vi "Arduino_DHT22_sensor.vi"() -> ()   [LabVIEW 2013]
uses:
  <vilib>/Instr/_visa.llb/VISA Configure Serial Port (Instr).vi
panel:
  out "Waveform Chart 2":dbl[](graph)
  out "Dew Point Temp (C)":dbl
  out "Temp (C)":dbl
  out "Waveform Chart":dbl[](graph)
  out "Humidity (%)":dbl
  in  "stop":bool
  # "Arduino Temperature and Humidity Sensing"
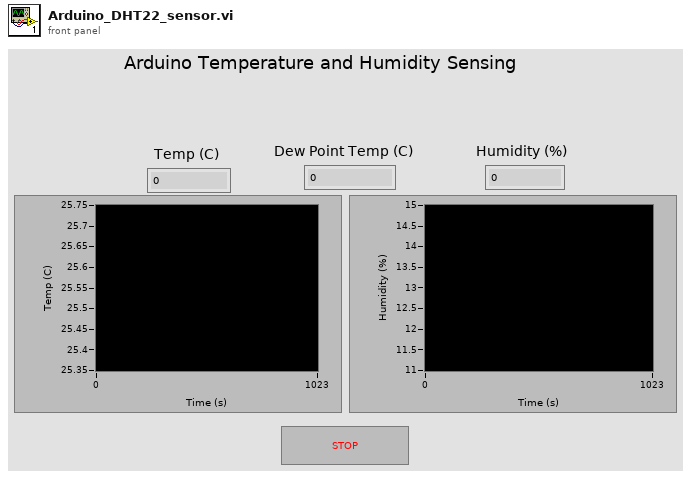
[diagram p1: front panel]
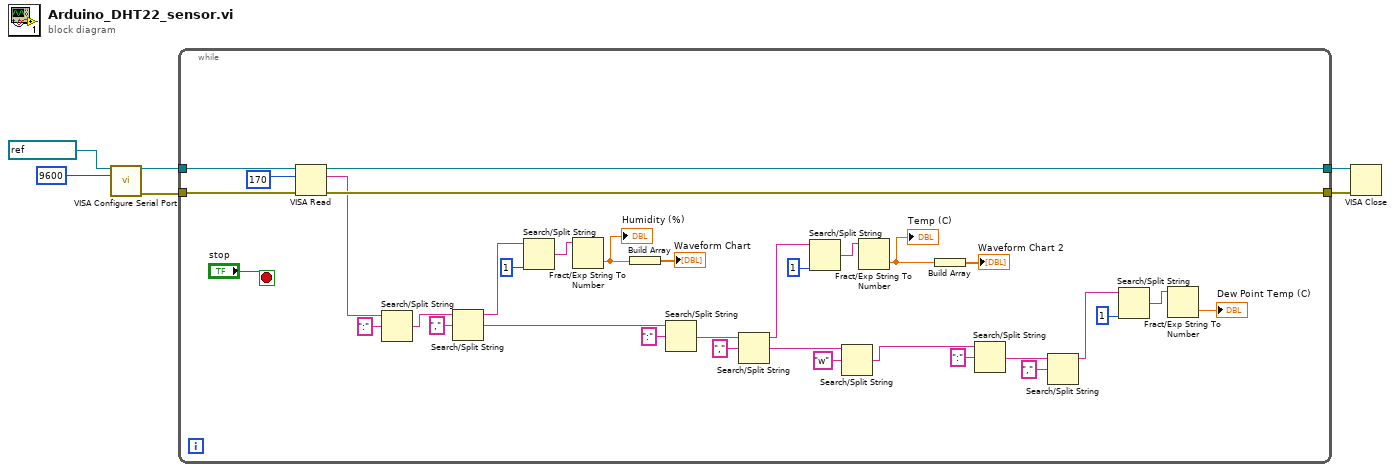
[diagram p0: block diagram]
diagram:
  n1 = call-poly "VISA Configure Serial Port"("VISA resource name"=refnum<visa-resource-name> "COM12", "baud rate (9600)"=u32 9600) -> ("VISA resource name out"=w3:refnum<visa-resource-name>, "error out"=w4:errorcluster)  [unwired: 12 in]
  n2 = while {
    tunnel: w3 -> [w36]
    tunnel: w4 -> [w35]
    tunnel: [w39] -> w6
    tunnel: [w38] -> w5
    stop <- "stop" stop-if-true
    n3 = VISA Read(VISA resource name=w36, byte count=u32 170, error in (no error)=w35) -> (VISA resource name out=w39:refnum<visa-resource-name>, read buffer=w34:string, error out=w38:errorcluster)  [unwired: 1 out]
    n4 = Search/Split String(string=w34, search string/char (-)=":") -> (match + rest of string=w31:string)  [unwired: 1 in, 2 out]
    n5 = Search/Split String(string=w31, search string/char (-)=",") -> (substring before match=w26:string, match + rest of string=w30:string)  [unwired: 1 in, 1 out]
    n6 = Search/Split String(string=w26, offset (0)=1) -> (match + rest of string=w24:string)  [unwired: 1 in, 2 out]
    n7 = Fract/Exp String To Number(string=w24) -> (number=w23:dbl)  [unwired: 3 in, 1 out]
    "Humidity (%)" <- w23
    n8 = Build Array(w23) -> (→"Waveform Chart":dbl[])
    n9 = Search/Split String(string=w30, search string/char (-)=":") -> (match + rest of string=w27:string)  [unwired: 1 in, 2 out]
    n10 = Search/Split String(string=w27, search string/char (-)=",") -> (substring before match=w18:string, match + rest of string=w10:string)  [unwired: 1 in, 1 out]
    n11 = Search/Split String(string=w18, offset (0)=1) -> (match + rest of string=w20:string)  [unwired: 1 in, 2 out]
    n12 = Search/Split String(string=w10, search string/char (-)="w") -> (match + rest of string=w9:string)  [unwired: 1 in, 2 out]
    n13 = Fract/Exp String To Number(string=w20) -> (number=w21:dbl)  [unwired: 3 in, 1 out]
    "Temp (C)" <- w21
    n14 = Build Array(w21) -> (→"Waveform Chart 2":dbl[])
    n15 = Search/Split String(string=w9, search string/char (-)=":") -> (match + rest of string=w14:string)  [unwired: 1 in, 2 out]
    n16 = Search/Split String(string=w14, search string/char (-)=",") -> (substring before match=w17:string)  [unwired: 1 in, 2 out]
    n17 = Search/Split String(string=w17, offset (0)=1) -> (match + rest of string=w15:string)  [unwired: 1 in, 2 out]
    n18 = Fract/Exp String To Number(string=w15) -> (number=→"Dew Point Temp (C)":dbl)  [unwired: 3 in, 1 out]
  }
  n19 = VISA Close(VISA resource name=w6, error in (no error)=w5) -> ()  [unwired: 1 out]
